vi "EminemNetworkingGlobal.vi"() -> ()   [LabVIEW 2023]
panel:
  in  "BoxState":string
  out "BoxReady":bool
  out "ShooterSensor":bool
  out "IntakeSensor":bool
  in  "RShooterMotorOutput":dbl
  in  "LShooterMotorOutput":dbl
  out "RAtSpeed":bool
  out "LAtSpeed":bool
  in  "RShooterFilteredSpeed":dbl
  in  "RShooterSpeed":dbl
  in  "LShooterFilteredSpeed":dbl
  in  "LShooterSpeed":dbl
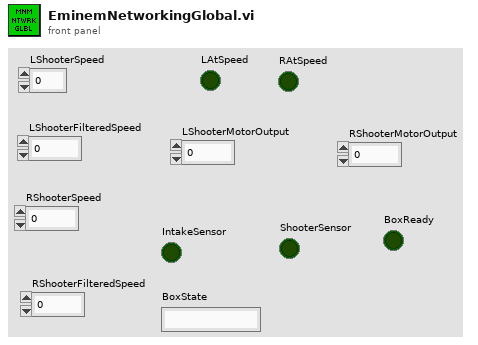
[diagram p1: front panel]
diagram:
